vi "Configure Status Questionable Ptransition.vi"(8 "error in":errorcluster, 9 "Value":u16 max=255, 11 "VISA resource name":refnum<visa-resource-name>) -> (0 "error out":errorcluster, 3 "VISA resource name out":refnum<visa-resource-name>)   [LabVIEW 2015, in "IT-M7700.lvlib"]
doc: "This command edits the value of the query forward jump trigger register.\n<b>Value</b>\n0-255"
uses:
  <instrlib>/IT-M7700/IT-M7700.lvlib
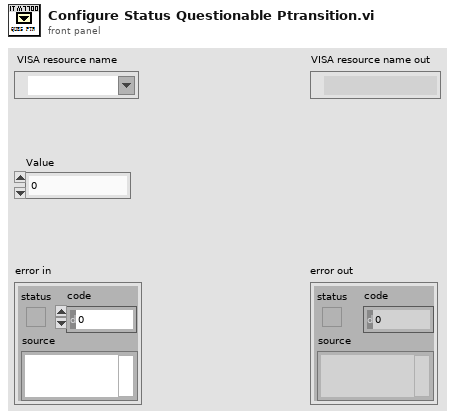
[diagram p1: front panel]
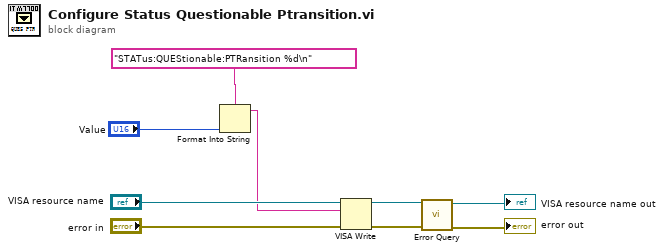
[diagram p0: block diagram]
diagram:
  n1 = Format Into String(format string="STATus:QUEStionable:PTRansition %d\n", "Value") -> (resulting string=w6:string)  [unwired: 2 in, 1 out]
  n2 = VISA Write(VISA resource name="VISA resource name", write buffer=w6, error in (no error)="error in") -> (VISA resource name out=w4:refnum<visa-resource-name>, error out=w3:errorcluster)  [unwired: 1 out]
  n3 = call <instrlib>:"Error Query.vi"("error in"=w3, "VISA resource name"=w4) -> ("error out"=→"error out":errorcluster, "VISA resource name out"=→"VISA resource name out":refnum<visa-resource-name>)  [unwired: 6 in, 2 out]
